vi "SpinEchoAmplitudeExtraction(SubVI).vi"(10 "Pulse Train File in":path, 11 "Larmor Frequency in":dbl=27410000.0 caption="Frequency" format="%.4p") -> (1 "Y value":dbl format="%0.2f", 2 "Signal Intensity (Integral)":dbl=0.6544283602926818 format="%0.4f", 3 "Extracted T2 Decay - Current Scan":waveform(dbl)(graph)={"t0"=timestamp(0 s since 1904-01-01), "dt"=0.0012610340479192938, "Y"=array[3965 elements]} caption="Waveform Graph", 4 "Larmor Frequency 3":dbl, 5 "Pulse Echos - Current Scan":waveform(dbl)(graph)={"t0"=timestamp(0 s since 1904-01-01), "dt"=0.0012610340479192938, "Y"=array[3965 elements]} caption="Waveform Graph")   [LabVIEW 2020]
uses:
  <instrlib>/niFgen/niFgen.llb/niFgen Waveform Type.ctl
  <instrlib>/niFgen/niFgen.llb/niFgen_ctl Trigger DigEdge - Edge Values (Ring).ctl
  <instrlib>/niFgen/niFgen.llb/niFgen_ctl Trigger Source Values (Ring).ctl
  <instrlib>/niFgen/niFgen.llb/niFgen Trigger Mode.ctl
  <instrlib>/niScope/Controls/niScope acquisition type.ctl
  <instrlib>/niScope/Controls/niScope trigger slope.ctl
  <instrlib>/niScope/Controls/niScope trigger source.ctl
  <vilib>/Analysis/2dsp.llb/Integral Method.ctl
  <instrlib>/niFgen/niFgen.llb/niFgen Output Mode.ctl
  <vilib>/Analysis/8numeric.llb/1D Numeric Integration.vi
  <instrlib>/niScope/Configure/Trigger/niScope Configure Trigger Edge.vi
  <instrlib>/niFgen/niFgen.llb/niFgen Configure Digital Edge Start Trigger.vi
  <instrlib>/niScope/Acquire/Fetch/niScope Fetch Cluster.vi
  <vilib>/Utility/file.llb/Read Delimited Spreadsheet (DBL).vi
  <instrlib>/niFgen/niFgen.llb/niFgen Create Waveform (DBL).vi
  <vilib>/Waveform/WDTOps.llb/WDT Get XY Value DBL.vi
  <vilib>/Analysis/NI_AALPro.lvlib
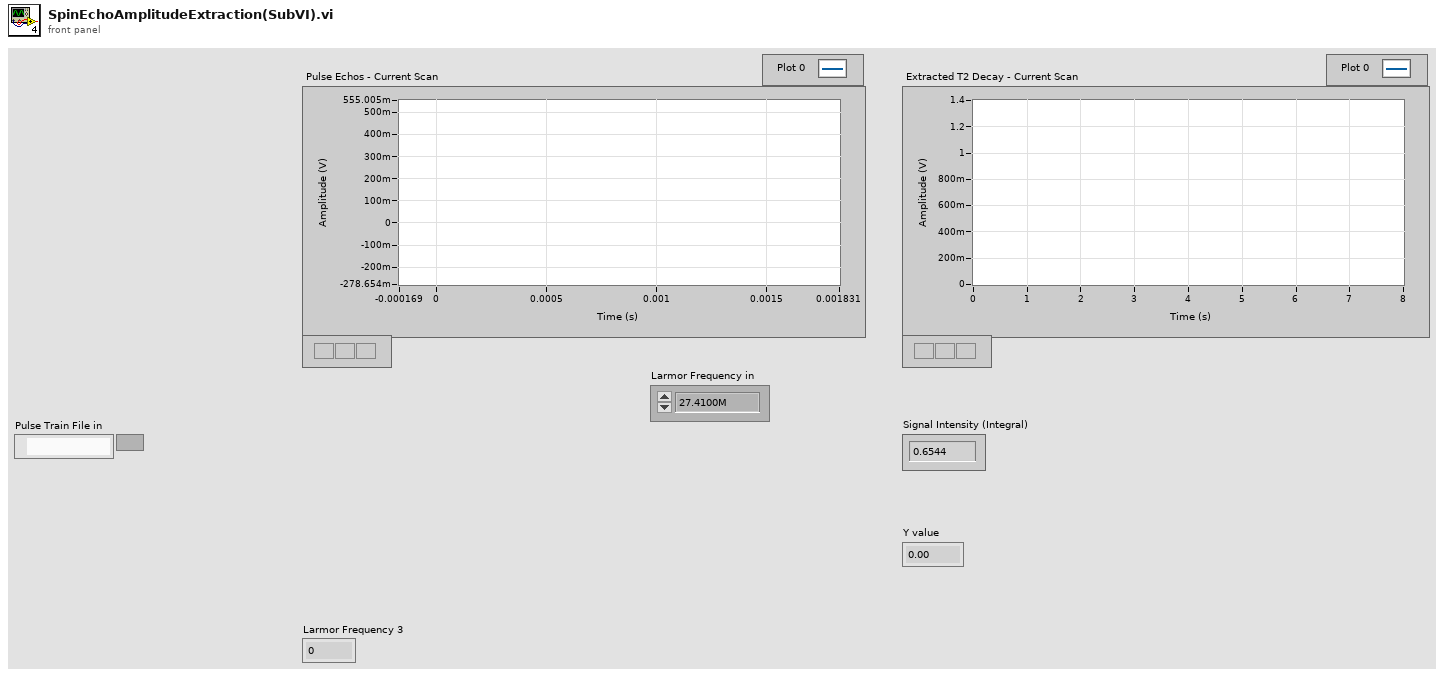
[diagram p1: front panel]
types:
  T1 = typedef "niFgen Output Mode.ctl" = u32
  T2 = typedef "NI_AALPro.lvlib/Integral Method.ctl" = i32
  T3 = typedef "niScope trigger source.ctl" = string
  T4 = typedef "niScope trigger slope.ctl" = i32
  T5 = typedef "niScope acquisition type.ctl" = i32
  T6 = typedef "niFgen Trigger Mode.ctl" = i32
  T7 = typedef "niFgen_ctl Trigger Source Values (Ring).ctl" = string
  T8 = typedef "niFgen_ctl Trigger DigEdge - Edge Values (Ring).ctl" = i32
  T9 = typedef "niFgen Waveform Type.ctl" = i32
  T10 = cluster{"relativeInitialX":dbl, "xIncrement":dbl, "wfm":dbl[]}
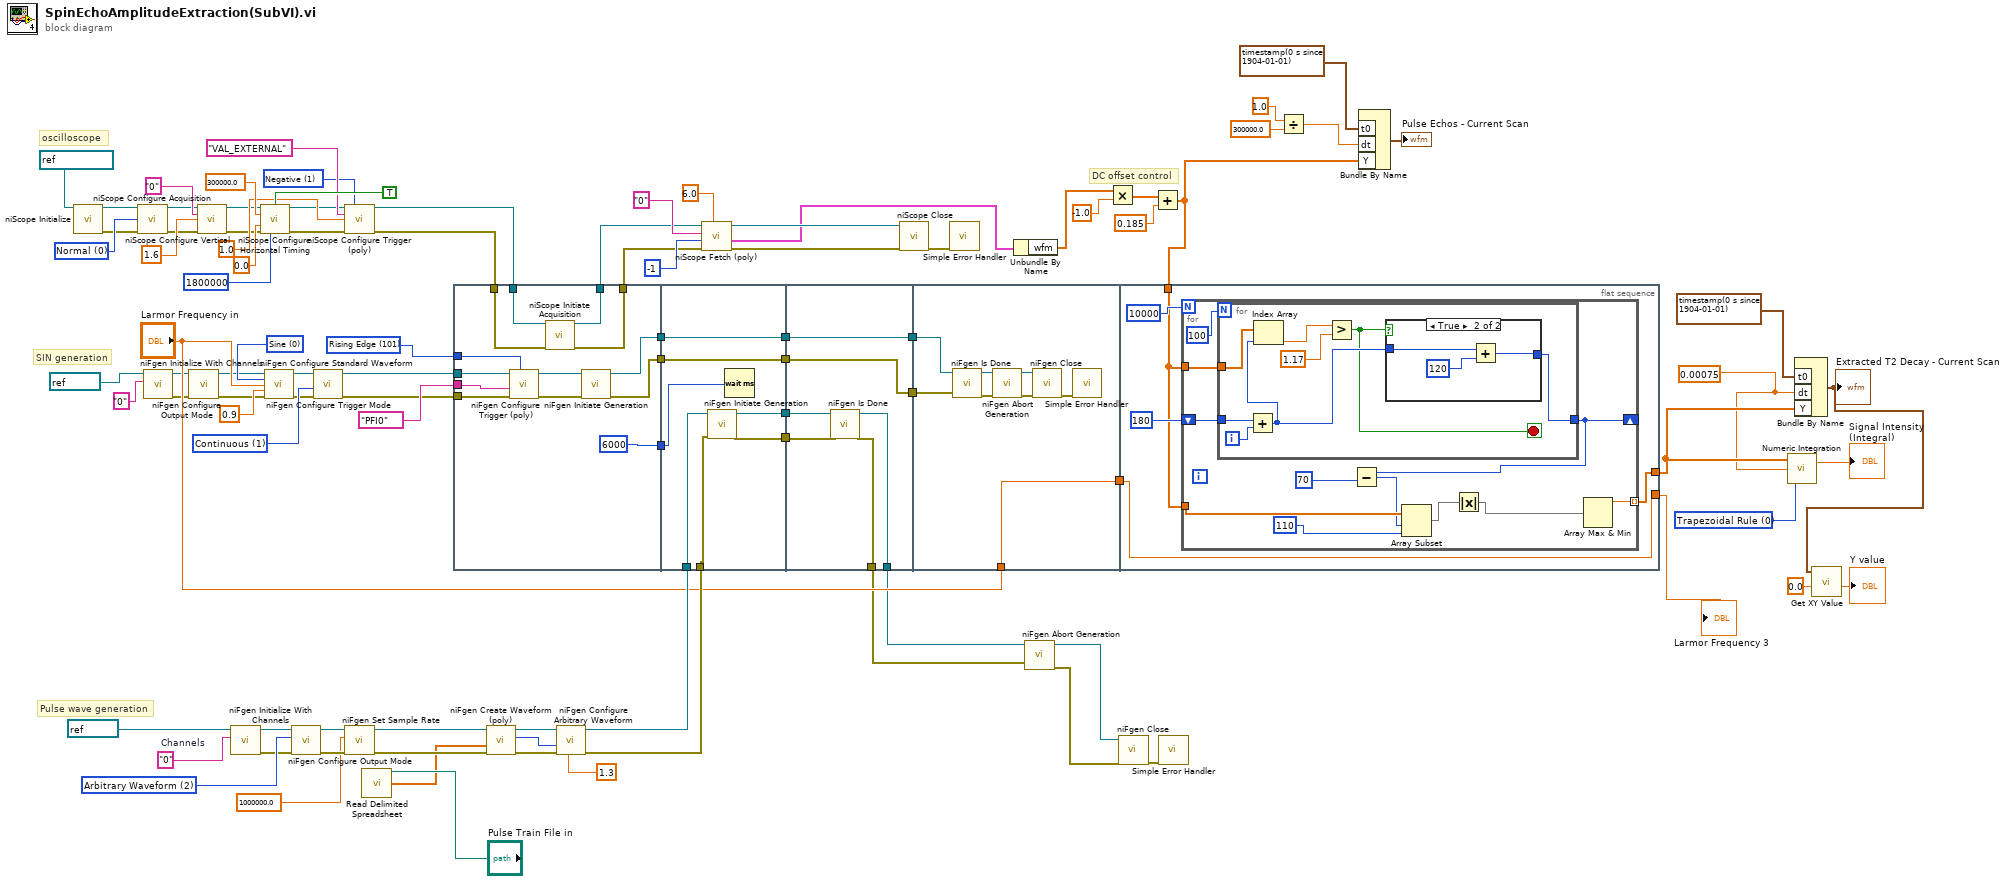
[diagram p0: block diagram]
diagram:
  w2 = 0.00075 ("dt")
  w17 = "0"  # Channels
  w18 = T1 2 items=["Standard Function", "Frequency List", "Arbitrary Waveform", "Arbitrary Sequence", "Script"] ("output mode")
  w63 = T2 0 items=["Trapezoidal Rule", "Simpson's Rule", "Simpson's 3/8 Rule", "Bode Rule"] ("integration method")
  w47 = T4 1 items=["Positive", "Negative"] ("trigger slope")
  w46 = T5 0 items=["Normal"=0, "Flex Res"=1, "DDC"=3] ("acquisition Type")
  w33 = T6 1 items=["Single", "Continuous", "Stepped", "Burst"] ("Trigger Mode (default: 1=continuous)")
  w29 = T8 101 items=["Rising Edge"=101, "Falling Edge"=102] ("Edge (Rising)")
  w28 = T9 0 items=["Sine", "Square", "Triangle", "Ramp Up", "Ramp Down", "DC", "Noise", "User"] ("Waveform")
  # "Pulse wave generation"
  # "SIN generation"
  # "oscilloscope"
  # "DC offset control"
  n1 = call <instrlib>:"niScope Initialize.vi"("resource name"=refnum<k15> "PXI1Slot2") -> ("instrument handle"=w45:refnum<k15>, "error out"=w44:errorcluster)  [unwired: 13 in]
  n2 = call <instrlib>:"niScope Configure Acquisition.vi"("instrument handle"=w45, "acquisition Type"=w46, "error in"=w44) -> ("instrument handle out"=w42:refnum<k15>, "error out"=w41:errorcluster)  [unwired: 11 in]
  n3 = call <instrlib>:"niFgen Initialize With Channels.vi"("Channel Name"="0", "Resource Name"=refnum<k15> "Dev2" ("Sine Wave Module")) -> ("error out"=w23:errorcluster, "Instrument Handle Out"=w20:refnum<k15>)  [unwired: 8 in]
  n4 = call <instrlib>:"niFgen Configure Output Mode.vi"("error in (no error)"=w23, "Instrument Handle"=w20) -> ("error out"=w24:errorcluster, "Instrument Handle Out"=w21:refnum<k15>)  [unwired: 7 in]
  n5 = call <instrlib>:"niScope Configure Vertical.vi"("instrument handle"=w42, "channels"="0", "vertical range"=1.6, "error in"=w41) -> ("instrument handle out"=w40:refnum<k15>, "error out"=w39:errorcluster)  [unwired: 10 in]
  n6 = call <instrlib>:"niFgen Initialize With Channels.vi"("Channel Name"=w17, "Resource Name"=refnum<k15> "Dev1" ("FGEN Resource Name 2")) -> ("error out"=w14:errorcluster, "Instrument Handle Out"=w13:refnum<k15>)  [unwired: 8 in]
  n7 = call <instrlib>:"niScope Configure Horizontal Timing.vi"("instrument handle"=w40, "enforce realtime"=TRUE, "min sample rate"=300000.0, "reference position"=0.0, "error in"=w39, "min record length"=1800000) -> ("instrument handle out"=w38:refnum<k15>, "error out"=w37:errorcluster)  [unwired: 8 in]
  n8 = call <instrlib>:"niFgen Configure Standard Waveform.vi"("Instrument Handle"=w21, "Waveform"=w28, "Frequency"="Larmor Frequency in", "Amplitude"=0.9, "error in (no error)"=w24) -> ("Instrument Handle Out"=w22:refnum<k15>, "error out"=w25:errorcluster)  [unwired: 9 in]
  n9 = call <instrlib>:"niFgen Configure Output Mode.vi"("error in (no error)"=w14, "Output Mode (default: 0=Standard Function)"=w18, "Instrument Handle"=w13) -> ("error out"=w10:errorcluster, "Instrument Handle Out"=w11:refnum<k15>)  [unwired: 6 in]
  n10 = call <instrlib>:"niFgen Configure Trigger Mode.vi"("error in (no error)"=w25, "Trigger Mode (default: 1=continuous)"=w33, "Instrument Handle"=w22) -> ("error out"=w30:errorcluster, "Instrument Handle Out"=w32:refnum<k15>)  [unwired: 7 in]
  n11 = call-poly <instrlib>:"niScope Configure Trigger (poly).vi"("instrument handle"=w38, "trigger slope"=w47, "trigger source"=T3 "VAL_EXTERNAL", "trigger level"=1.0, "error in"=w37) -> ("instrument handle out"=w53:refnum<k15>, "error out"=w54:errorcluster)  [unwired: 9 in]
  n12 = call <instrlib>:"niFgen Set Sample Rate.vi"("error in (no error)"=w10, "Sample Rate (Samp/s)"=1000000.0 ("Sample Rate"), "Instrument Handle"=w11) -> ("error out"=w7:errorcluster, "Instrument Handle Out"=w8:refnum<k15>)  [unwired: 7 in]
  n13 = call-poly <vilib>:"Read Delimited Spreadsheet.vi"("file path (dialog if empty)"="Pulse Train File in") -> ("first row"=w6:dbl[])  [unwired: 9 in, 5 out]
  n14 = flat-sequence {
    tunnel: w29 -> [w110]
    tunnel: w30 -> [w109]
    tunnel: T7 "PFI0" ("Source") -> [w108]
    tunnel: w32 -> [w107]
    tunnel: w53 -> [w105]
    tunnel: w54 -> [w104]
    tunnel: [w103] -> w55
    tunnel: [w102] -> w56
    tunnel: [w101] -> w98
    tunnel: [w100] -> w97
    tunnel: [u32 6000 ("milliseconds to wait")] -> w1
    tunnel: [w118] -> w96
    tunnel: [w117] -> w95
    tunnel: [w116] -> w94
    tunnel: w98 -> [w116]
    tunnel: [w115] -> w93
    tunnel: w97 -> [w115]
    tunnel: w86 -> [w114]
    tunnel: w87 -> [w113]
    tunnel: w1 -> [w112]
    tunnel: [w124] -> w34
    tunnel: [w123] -> w35
    tunnel: w96 -> [w122]
    tunnel: w95 -> [w121]
    tunnel: [w120] -> w92
    tunnel: w94 -> [w120]
    tunnel: [w119] -> w91
    tunnel: w93 -> [w119]
    tunnel: w92 -> [w127]
    tunnel: w91 -> [w126]
    tunnel: "Larmor Frequency in" -> [w125]
    tunnel: [w125] -> w90
    tunnel: w80 -> [w134]
    tunnel: [w136] -> w70
    tunnel: [w133] -> w85
    tunnel: w90 -> [w133]
    frame #0 {
      n15 = call-poly <instrlib>:"niFgen Configure Trigger (poly).vi"("Edge (Rising)"=w110, "error in (no error)"=w109, "Source"=w108, "Instrument Handle"=w107) -> ("error out"=w106:errorcluster, "Instrument Handle Out"=w111:refnum<k15>)  [unwired: 6 in]
      n16 = call <instrlib>:"niScope Initiate Acquisition.vi"("instrument handle"=w105, "error in"=w104) -> ("instrument handle out"=w103:refnum<k15>, "error out"=w102:errorcluster)  [unwired: 12 in]
      n17 = call <instrlib>:"niFgen Initiate Generation.vi"("error in (no error)"=w106, "Instrument Handle"=w111) -> ("error out"=w100:errorcluster, "Instrument Handle Out"=w101:refnum<k15>)  [unwired: 8 in]
    }
    frame #1 {
      n18 = call <instrlib>:"niFgen Initiate Generation.vi"("error in (no error)"=w114, "Instrument Handle"=w113) -> ("error out"=w117:errorcluster, "Instrument Handle Out"=w118:refnum<k15>)  [unwired: 8 in]
      n19 = Wait (ms)(milliseconds to wait=w112) -> ()  [unwired: 1 out]
    }
    frame #2 {
      n20 = call <instrlib>:"niFgen Is Done.vi"("error in (no error)"=w121, "Instrument Handle"=w122) -> ("error out"=w124:errorcluster, "Instrument Handle Out"=w123:refnum<k15>)  [unwired: 7 in, 1 out]
    }
    frame #3 {
      n21 = call <instrlib>:"niFgen Is Done.vi"("error in (no error)"=w126, "Instrument Handle"=w127) -> ("error out"=w130:errorcluster, "Instrument Handle Out"=w129:refnum<k15>)  [unwired: 7 in, 1 out]
      n22 = call <instrlib>:"niFgen Abort Generation.vi"("error in (no error)"=w130, "Instrument Handle"=w129) -> ("error out"=w131:errorcluster, "Instrument Handle Out"=w132:refnum<k15>)  [unwired: 8 in]
      n23 = call <instrlib>:"niFgen Close.vi"("error in (no error)"=w131, "Instrument Handle"=w132) -> ("error out"=w128:errorcluster)  [unwired: 9 in]
      n24 = call <vilib>:"Simple Error Handler.vi"("error in (no error)"=w128) -> ()  [unwired: 4 in, 5 out]
    }
    frame #4 {
      n25 = for {
        N: 10000 -> [_]
        tunnel: [w148] -> w136 mode=indexing
        tunnel: w134 -> [w147]
        shift-right: [w143] -> _
        shift-left: 180 -> [w146]
        tunnel: w134 -> [w145]
        n26 = for {
          N: 100 -> [_]
          tunnel: w145 -> [w152]
          tunnel: w146 -> [w155]
          tunnel: [w150] -> w143
          i -> [w156]
          stop <- w149 stop-if-true
          n27 = Add(x=w155, y=w156) -> (x+y=w151:i32)
          n28 = Index Array(array=w152, index=w151) -> (element=w153:dbl)
          n29 = Greater?(x=w153, y=1.17) -> (0:w149:bool)
          n30 = case shown="True" w149 {
            tunnel: w151 -> [w157 w158]
            tunnel: [w157 w160] -> w150
            frame False {
            }
            frame True {
              n31 = Add(x=w158, y=120) -> (x+y=w160:i32)
            }
          }
        }
        n32 = Subtract(x=w143, y=70) -> (x-y=w141:i32)
        n33 = Array Subset(array=w147, index=w141, length=110 ("y")) -> (w139:dbl[])
        n34 = Absolute Value(x=w139) -> (abs(x)=w138:dbl[])
        n35 = Array Max & Min(array=w138) -> (max value=w148:dbl)  [unwired: 3 out]
      }
    }
  }
  n36 = call-poly <instrlib>:"niFgen Create Waveform (poly).vi"("error in (no error)"=w7, "Waveform Data Array"=w6, "Instrument Handle"=w8) -> ("error out"=w4:errorcluster, "Waveform Handle"=w3:i32, "Instrument Handle Out"=w5:refnum<k15>)  [unwired: 6 in]
  n37 = call <instrlib>:"niFgen Configure Arbitrary Waveform.vi"("Gain"=1.3, "error in (no error)"=w4, "Waveform Handle"=w3, "Instrument Handle"=w5) -> ("error out"=w86:errorcluster, "Instrument Handle Out"=w87:refnum<k15>)  [unwired: 6 in]
  n38 = call-poly <instrlib>:"niScope Fetch (poly).vi"("timeout"=6.0, "error in"=w56, "numSamples"=-1, "channels"="0", "instrument handle"=w55) -> ("error out"=w68:errorcluster, "waveform"=w65:T10, "instrument handle out"=w67:refnum<k15>)  [unwired: 3 in, 1 out]
  n39 = call <instrlib>:"niScope Close.vi"("instrument handle"=w67, "error in"=w68) -> ("error out"=w36:errorcluster)  [unwired: 13 in]
  n40 = call <vilib>:"Simple Error Handler.vi"("error in (no error)"=w36) -> ()  [unwired: 4 in, 5 out]
  n41 = Unbundle By Name(w65) -> ("wfm"=w76:dbl[])
  n42 = call <instrlib>:"niFgen Abort Generation.vi"("error in (no error)"=w34, "Instrument Handle"=w35) -> ("error out"=w88:errorcluster, "Instrument Handle Out"=w89:refnum<k15>)  [unwired: 8 in]
  n43 = Multiply(x=w76, y=-1.0) -> (x*y=w79:dbl[])
  n44 = call <instrlib>:"niFgen Close.vi"("error in (no error)"=w88, "Instrument Handle"=w89) -> ("error out"=w19:errorcluster)  [unwired: 9 in]
  n45 = Add(x=w79, y=0.185) -> (x+y=w80:dbl[])
  n46 = call <vilib>:"Simple Error Handler.vi"("error in (no error)"=w19) -> ()  [unwired: 4 in, 5 out]
  n47 = Divide(x=1.0, y=300000.0) -> (x/y=w75:dbl)
  n48 = Bundle By Name("t0"=timestamp(0 s since 1904-01-01), "dt"=w75, "Y"=w80) -> (→"Pulse Echos - Current Scan":waveform(dbl))  [unwired: 1 in]
  n49 = call-poly <vilib>:"Numeric Integration.vi"("integration method"=w63, "dt"=w2, "Input Array"=w70) -> ("result"=→"Signal Intensity (Integral)":dbl)  [unwired: 1 out]
  n50 = Bundle By Name("t0"=timestamp(0 s since 1904-01-01), "dt"=w2, "Y"=w70) -> (w81:waveform(dbl))  [unwired: 1 in]
  "Extracted T2 Decay - Current Scan" <- w81
  n51 = call-poly <vilib>:"Get XY Value.vi"("Y position"=0.0, "waveform in"=w81) -> ("Y value"=→"Y value":dbl)  [unwired: 5 in, 4 out]
  "Larmor Frequency 3" <- w85
